vi "Lock DB.vi"(8 "error in (no error)":errorcluster, 10 "Lock?":bool, 11 "Simulated Configuration Database Actor in":refnum<class "Simulated Configuration Database Actor.lvclass">=refnum) -> (0 "error out":errorcluster, 3 "Simulated Configuration Database Actor out":refnum<class "Simulated Configuration Database Actor.lvclass">)   [LabVIEW 2019, in "Sim Configuration Database Actor.lvlib" / "Sim Configuration Database Actor.lvclass"]
uses:
  Sim Configuration Database Actor.lvclass
  Simulated Configuration Database Actor/Simulated Configuration Database Actor/Configuration Database Actor.lvclass
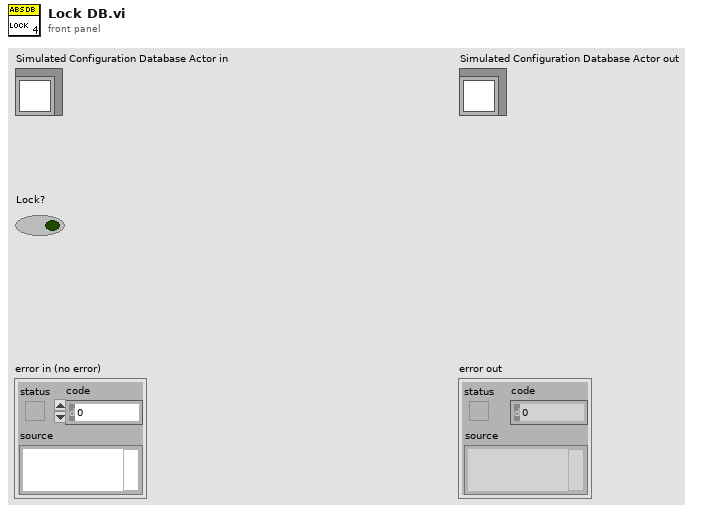
[diagram p1: front panel]
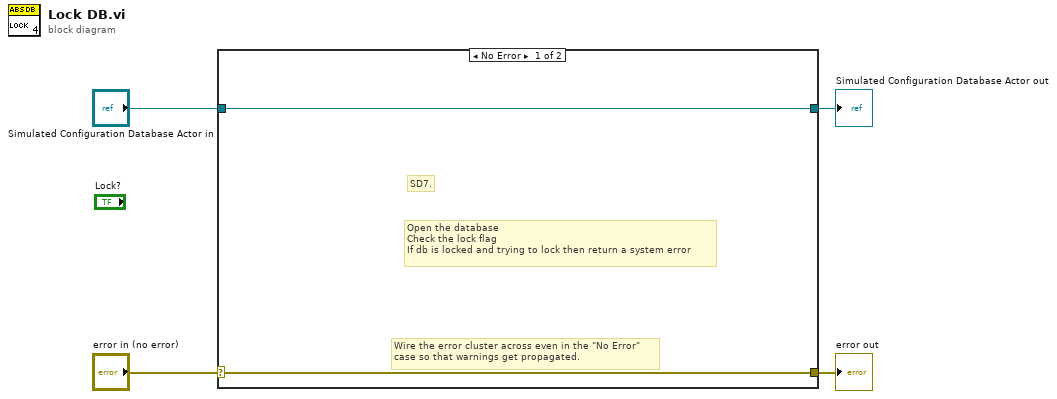
[diagram p0: block diagram]
diagram:
  n1 = case shown="No Error" "error in (no error)" {
    selector: "error in (no error)" -> [w5 w8]
    tunnel: [w5 w8] -> w3
    tunnel: [w6 w7] -> w1
    tunnel: "Simulated Configuration Database Actor in" -> [w6 w7]
    frame No Error {
      # "Open the database\nCheck the lock flag\nIf db is locked and trying to lock then return a system error"
      # "SD7."
      # "Wire the error cluster across even in the \"No Error\"\ncase so that warnings get propagated."
    }
    frame Error {
    }
  }
  "error out" <- w3
  "Simulated Configuration Database Actor out" <- w1
